vi "UDcluster to File.vi"(1 "User-data cluster":T1) -> (0 "CypheredText":string)   [LabVIEW 2012]
uses:
  typedef/User_Data_Cluster.ctl
  typedef/User Accounts.ctl
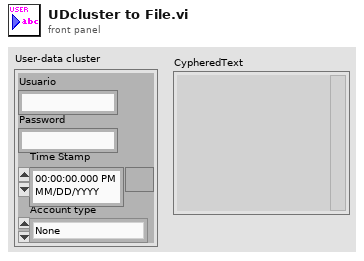
[diagram p1: front panel]
types:
  T1 = typedef "User_Data_Cluster.ctl" = cluster{"Usuario":string, "Password":string, "Account type":T2, "Time Stamp":timestamp}
  T2 = typedef "User Accounts.ctl" = enum16{"None", "User", "Admin"}
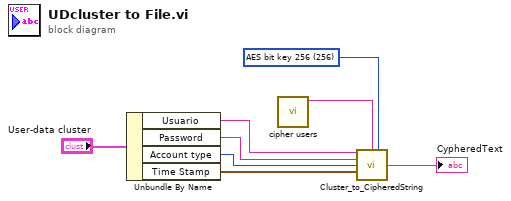
[diagram p0: block diagram]
diagram:
  w3 = u16 256 items=["AES bit key 128"=128, "AES bit key 192"=192, "AES bit key 256"=256] ("BitKeyType(256)")
  n1 = Unbundle By Name("User-data cluster") -> ("Usuario"=w7:string, "Password"=w6:string, "Account type"=w5:T2, "Time Stamp"=w4:timestamp)
  n2 = call "cipher users.vi"() -> ("password to cipher users"=w2:string)  [unwired: 11 in]
  n3 = call "Cluster_to_CipheredString.vi"("Usuario"=w7, "password to cipher users"=w2, "BitKeyType(256)"=w3, "Actions"=w6, "Account type"=w5, "Time Stamp"=w4) -> ("CypheredText"=→"CypheredText":string)  [unwired: 8 in, 1 out]
